vi "Recieve.vi"(8 "error in (no error)":errorcluster, 9 "timeout in ms (-1)":i32=-1, 11 "Get Controls in":refnum<class "Get Controls.lvclass">) -> (0 "error out":errorcluster, 1 "Success?":bool, 3 "Control Element Array":T1[](array[typedef]))   [LabVIEW 2020, in "Msg.lvlib" / "Get Controls.lvclass"]
doc: "Recieve data from the queue and release the queue afterwards."
uses:
  Get Controls.lvclass
  Controls/Ctl_Control Element.ctl
  Get Controls.lvclass/Get Controls.ctl
  Msg.lvlib
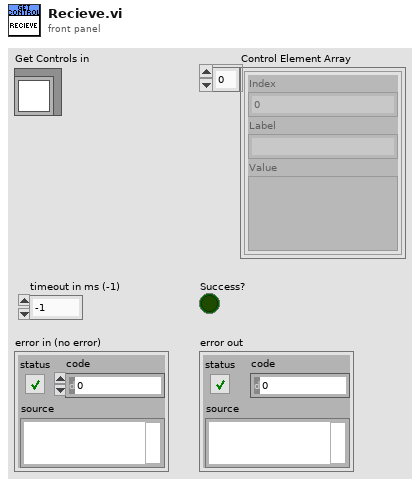
[diagram p1: front panel]
types:
  T1 = typedef "Msg.lvlib/Ctl_Control Element.ctl" = cluster{"Index":i32, "Label":string, "Value":variant}
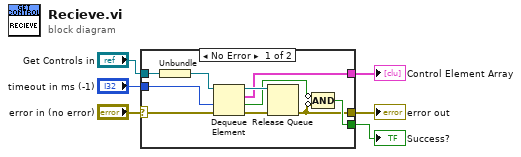
[diagram p0: block diagram]
diagram:
  n1 = case shown="No Error" "error in (no error)" {
    selector: "error in (no error)" -> [w11 w17]
    tunnel: "Get Controls in" -> [w16 _]
    tunnel: "timeout in ms (-1)" -> [w14 _]
    tunnel: [w12 _] -> w4
    tunnel: [w8 _] -> w2
    tunnel: [w7 w17] -> w1
    frame No Error {
      n2 = Unbundle(w16) -> (w15:refnum<queue>)
      n3 = Dequeue Element(queue=w15, timeout in ms (-1)=w14, error in (no error)=w11) -> (queue out=w13:refnum<queue>, element=w12:T1[], timed out?=w9:bool, error out=w10:errorcluster)
      n4 = Release Queue(queue=w13, error in (no error)=w10) -> (error out=w7:errorcluster)  [unwired: 1 in, 2 out]
      n5 = Compound Arithmetic op=AND(invert w9, invert w7) -> (w8:bool)
    }
    frame Error {
    }
  }
  "error out" <- w1
  "Control Element Array" <- w4
  "Success?" <- w2
